vi "_Serial Read Bit.vi"(1 "Port type":u8) -> (0 "BitState":bool)   [LabVIEW 2012]
uses:
  <vilib>/rvi/eio/common/nirviEmuTemplateMethod_errors.vi
  <vilib>/eio/EIONode/EIONode.xnode
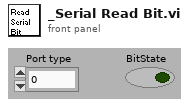
[diagram p1: front panel]
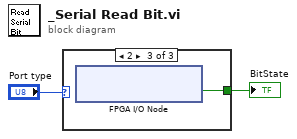
[diagram p0: block diagram]
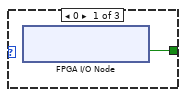
[diagram p2: hidden frame]
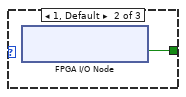
[diagram p3: hidden frame]
diagram:
  n1 = case shown="2" "Port type" {
    tunnel: [w3 w4 w5] -> w2
    frame 0 {
      n2 = xnode "FPGA I/O Node"() -> ("Digtal IO/DIO46"=w3:bool)  [unwired: 1 in, 1 out]
    }
    frame 1, Default {
      n3 = xnode "FPGA I/O Node"() -> ("Digtal IO/DIO44"=w4:bool)  [unwired: 1 in, 1 out]
    }
    frame 2 {
      n4 = xnode "FPGA I/O Node"() -> ("Digtal IO/DIO54"=w5:bool)  [unwired: 1 in, 1 out]
    }
  }
  "BitState" <- w2
